vi "generate default line.vi"(8 "error in":errorcluster, 11 "operations table":T2) -> (0 "error out":errorcluster, 2 "line":T1)   [LabVIEW 2013, in "Shared Library Module editor node.lvclass"]
doc: "Platypus Framework 1.0.1.60\nNI Systems Engineering - National Instruments"
uses:
  Shared Library Module editor node.lvclass
  table reference.ctl
  table line.ctl
  <vilib>/NI/Tag Bus Module Framework/channel/TBM channel.lvclass
  <vilib>/NI/Tag Bus/tag/Data Type.ctl
  permissions.ctl
  <vilib>/NI/Tag Bus/tag/tag descriptor.lvclass/tag descriptor.ctl
  <vilib>/NI/Tag Bus/tag/tag descriptor.lvclass
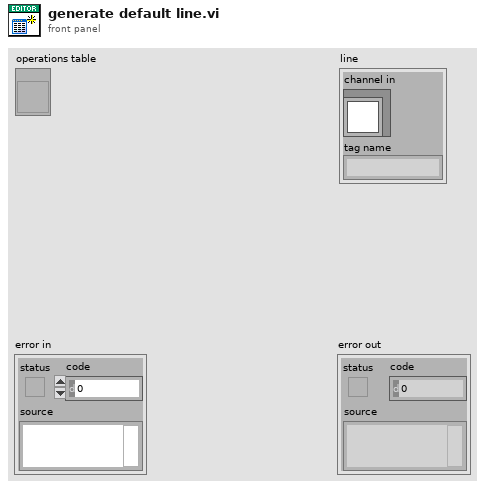
[diagram p1: front panel]
types:
  T1 = typedef "Shared Library Module editor node.lvclass/table line.ctl" = cluster{"channel in":refnum<class "TBM channel.lvclass">, "tag name":string}
  T2 = typedef "Shared Library Module editor node.lvclass/table reference.ctl" = refnum<vi>
  T3 = typedef "Shared Library Module editor node.lvclass/permissions.ctl" = enum32{"Processing Parameter", "Proecessing Result", "Input from Library", "Output to Library"}
  T4 = typedef "tag bus.lvlib/tag descriptor.lvclass/Data Type.ctl" = enum16{"Double", "Single", "I64", "I32", "I16", "I8", "U64", "U32", "U16", "U8", "Boolean", "String", "Array of Double", "Array of Single", "Array of I64", "Array of I32", "Array of I16", "Array of I8", "Array of U64", "Array of U32", "Array of U16", "Array of U8", "Array of Boolean", "Array of String"}
  T5 = typedef "TBM channel.lvclass/channel classification.ctl" = enum16{"input data", "output data", "processing parameter", "processing result"}
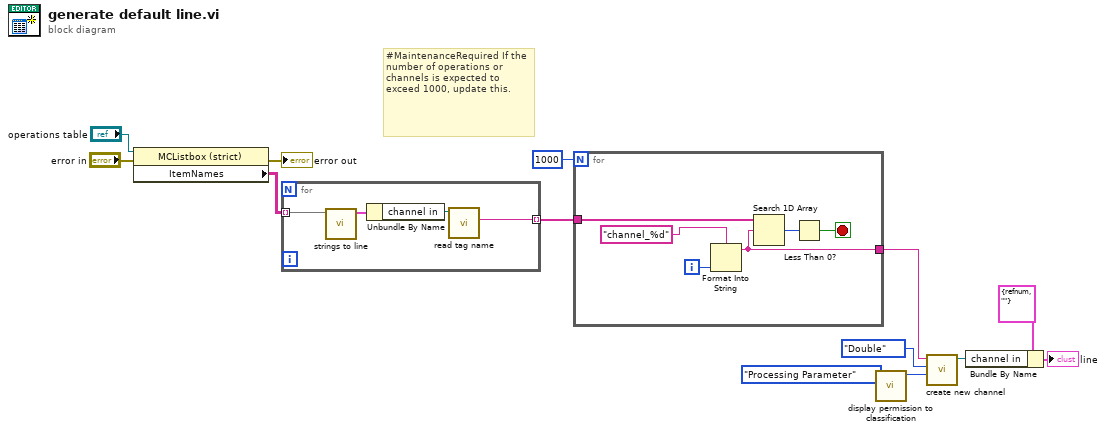
[diagram p0: block diagram]
diagram:
  # "#MaintenanceRequired If the number of operations or channels is expected to exceed 1000, update this."
  n1 = property class="MCListbox (strict)"(reference="operations table", error in="error in") -> (error out=→"error out":errorcluster, "ItemNames"=w10:string[][])  [unwired: 1 out]
  n2 = for {
    tunnel: w10 -> [w17] mode=indexing
    tunnel: [w14] -> w8 mode=indexing
    n3 = call "strings to line.vi"("strings"=w17) -> ("line"=w16:T1)  [unwired: 10 in]
    n4 = Unbundle By Name(w16) -> ("channel in"=w15:refnum<class "TBM channel.lvclass">)
    n5 = call <vilib>:"read tag name.vi"("system tag in"=w15) -> ("name"=w14:string)  [unwired: 8 in, 2 out]
  }
  n6 = for {
    N: 1000 -> [_]
    tunnel: w8 -> [w21]
    tunnel: [w18] -> w5
    i -> [w23]
    stop <- w19 stop-if-true
    n7 = Format Into String(format string="channel_%d", w23) -> (resulting string=w18:string)  [unwired: 2 in, 1 out]
    n8 = Search 1D Array(1D array=w21, element=w18) -> (index of element=w20:i32)  [unwired: 1 in]
    n9 = Less Than 0?(x=w20) -> (x < 0?=w19:bool)
  }
  n10 = call "display permission to classification.vi"("display permissions"=permissions."Processing Parameter") -> ("channel classification"=w1:T5)  [unwired: 10 in]
  n11 = call <vilib>:"create new channel.vi"("channel classification"=w1, "data type"=Data_Type."Double", "channel name"=w5) -> ("channel"=w4:refnum<class "TBM channel.lvclass">)  [unwired: 8 in]
  n12 = Bundle By Name(cluster=T1 {"channel in"=refnum, "tag name"=""} ("line"), "channel in"=w4) -> (→"line":T1)
